vi "VI Server - 호출자(엄격한).vi"() -> ()   [LabVIEW 2014]
uses:
  <vilib>/Analysis/4window.llb/windowTd.ctl
  <vilib>/measure/maspectr.llb/Power Spectrum and PSD Export Mode.ctl
  <vilib>/Analysis/NI_AALPro.lvlib
  <vilib>/measure/NI_MAPro.lvlib
panel:
  in  "export mode":T1 items=["파워 스펙트럼", "파워 스펙트럼 밀도"]
  in  "window":T2 items=["사각형"=0, "해닝"=1, "해밍"=2, "블랙맨-해리스"=3, "정밀한 블랙맨"=4, "블랙맨"=5, "플랫 탑(Flat Top)"=6, "4항 블랙맨-해리스 "=7, "7항 블랙맨-해리스"=8, "낮은 사이드로브"=9, "블랙맨 누탈"=11, "삼각파"=30, "바틀렛-해닝"=31, "보먼"=32, "파젠"=33, "웰치"=34, "카이저"=60, "돌프-체비셰프"=61, "가우스"=62]
  out "웨이브폼 그래프":cluster{"f0":dbl, "df":dbl, "magnitude":dbl[]}(graph)
  in  "dB On (F)":bool
  in  "Frequency":dbl
  out "에러 출력":errorcluster
  in  "vi 경로":path
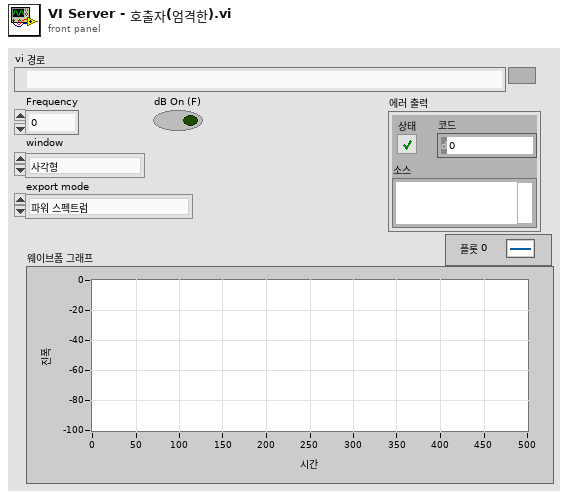
[diagram p1: front panel]
types:
  T1 = typedef "NI_MAPro.lvlib/Power Spectrum and PSD Export Mode.ctl" = u16
  T2 = typedef "NI_AALPro.lvlib/windowTd.ctl" = u32
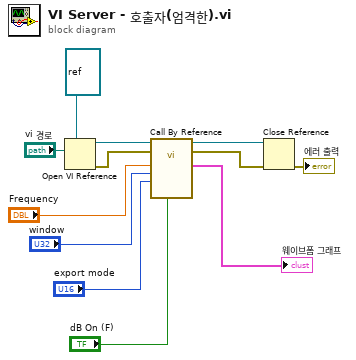
[diagram p0: block diagram]
diagram:
  n1 = Open VI Reference(type specifier VI Refnum (for type only)=refnum<vi> refnum ("타입 지정자 VI 참조 번호(타입만)"), vi path="vi 경로") -> (vi reference=w10:refnum<vi>, error out=w9:errorcluster)  [unwired: 4 in]
  n2 = call-by-ref "?"(reference=w10, error in=w9, "dB On (F)"="dB On (F)", "export mode"="export mode", "window"="window", "Frequency"="Frequency") -> (reference out=w8:refnum<vi>, error out=w7:errorcluster, "Power Spectrum / PSD"=→"웨이브폼 그래프":cluster{"f0":dbl, "df":dbl, "magnitude":dbl[]})  [unwired: 6 in, 1 out]
  n3 = Close Reference(reference=w8, error in (no error)=w7) -> (error out=→"에러 출력":errorcluster)
